vi "Create Mesh.vi"(8 "error in (no error)":errorcluster) -> (0 "error out":errorcluster, 3 "New Mesh Refnum":refnum<vi>)   [LabVIEW 2020, in "NI_3D Picture Control.lvlib"]
doc: "Creates a 3D mesh to apply to a 3D object that appears in a 3D scene."
uses:
  NI_3D Picture Control.lvlib
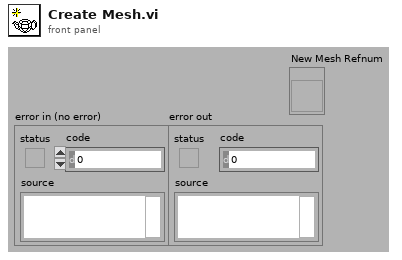
[diagram p1: front panel]
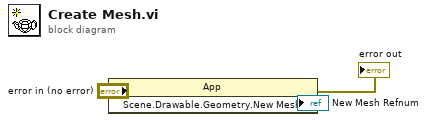
[diagram p0: block diagram]
diagram:
  n1 = invoke class="App" method="Scene.Drawable.Geometry.New Mesh"(error in="error in (no error)") -> (error out=→"error out":errorcluster, "Scene.Geometry.New Mesh"=→"New Mesh Refnum":refnum<vi>)  [unwired: 2 in, 1 out]
